vi "Create Build Events.vi"() -> (1 "Event Reg":refnum<event-registration>, 2 "Build Events":T1)   [LabVIEW 2020, in "Builder Tools.lvlib"]
uses:
  Builder/Builder.lvclass/Builder.ctl
  Builder Tools.lvlib
  Enable Cancel Data.ctl
  New Job Data.ctl
  New Item Data.ctl
  Complete Data.ctl
  Error Data.ctl
  Build Events.ctl
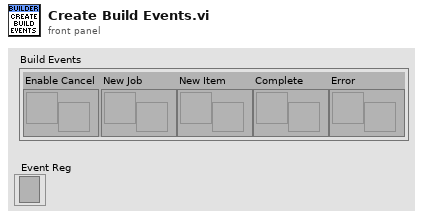
[diagram p1: front panel]
types:
  T1 = typedef "Builder Tools.lvlib/Build Events.ctl" = cluster{"Enable Cancel":refnum<user-event>, "New Job":refnum<user-event>, "New Item":refnum<user-event>, "Complete":refnum<user-event>, "Error":refnum<user-event>}
  T2 = typedef "Builder Tools.lvlib/Error Data.ctl" = cluster{"Message":string}
  T3 = typedef "Builder Tools.lvlib/Complete Data.ctl" = cluster{"Unused":bool}
  T4 = typedef "Builder Tools.lvlib/New Item Data.ctl" = cluster{"Message":string, "Progress":i32}
  T5 = typedef "Builder Tools.lvlib/New Job Data.ctl" = cluster{"Max Progress":i32}
  T6 = typedef "Builder Tools.lvlib/Enable Cancel Data.ctl" = cluster{"Unused":bool}
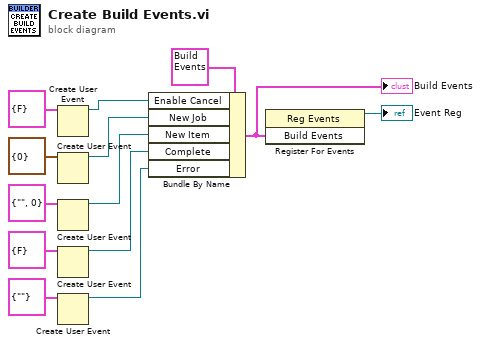
[diagram p0: block diagram]
diagram:
  n1 = Create User Event(user event datatype=T6 {"Unused"=FALSE} ("Enable Cancel Data")) -> (user event=w7:refnum<user-event>)  [unwired: 1 in, 1 out]
  n2 = Create User Event(user event datatype=T5 {"Max Progress"=0} ("New Job Data")) -> (user event=w6:refnum<user-event>)  [unwired: 1 in, 1 out]
  n3 = Create User Event(user event datatype=T4 {"Message"="", "Progress"=0} ("New Item Data")) -> (user event=w5:refnum<user-event>)  [unwired: 1 in, 1 out]
  n4 = Create User Event(user event datatype=T3 {"Unused"=FALSE} ("Complete Data")) -> (user event=w4:refnum<user-event>)  [unwired: 1 in, 1 out]
  n5 = Create User Event(user event datatype=T2 {"Message"=""} ("Error Data")) -> (user event=w3:refnum<user-event>)  [unwired: 1 in, 1 out]
  n6 = Bundle By Name(cluster=T1 {"Enable Cancel"=refnum, "New Job"=refnum, "New Item"=refnum, "Complete"=refnum, "Error"=refnum} ("Build Events"), "Enable Cancel"=w7, "New Job"=w6, "New Item"=w5, "Complete"=w4, "Error"=w3) -> (w2:T1)
  "Build Events" <- w2
  n7 = register-events(w2) -> (reference out=→"Event Reg":refnum<event-registration>)  [unwired: 2 in, 1 out]
